vi "notification location.vi"(3 "Bottom Right":bool, 4 "Bottom Left":bool, 5 "Top Right":bool, 6 "Top Left":bool) -> (0 "ButtonStates":bool[](array[boolean]), 1 "Text Justification":enum16{"Left", "Center", "Right"}(ring), 2 "Position":T1)   [LabVIEW 2015]
uses:
  <vilib>/Utility/miscctls.llb/LVPositionTypeDef.ctl
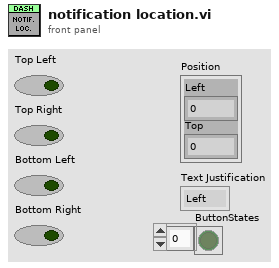
[diagram p1: front panel]
types:
  T1 = typedef "LVPositionTypeDef.ctl" = cluster{"Left":i32, "Top":i32}
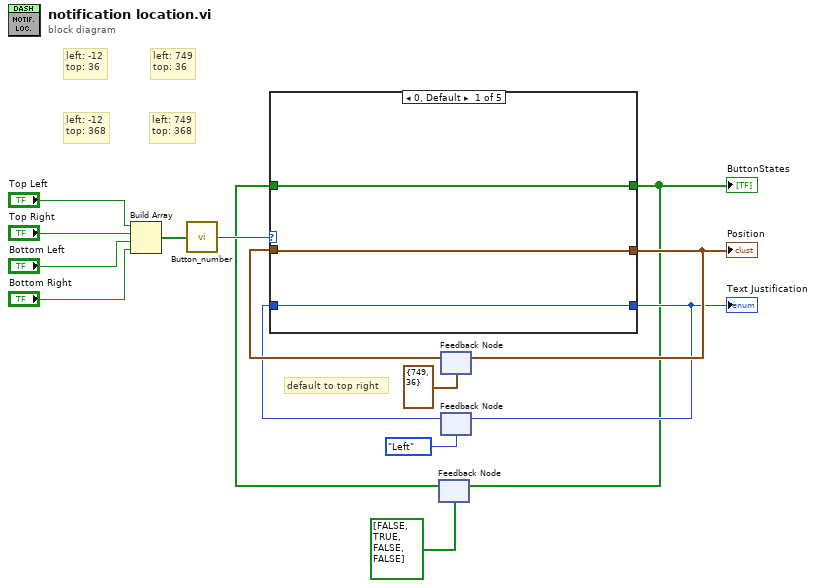
[diagram p0: block diagram]
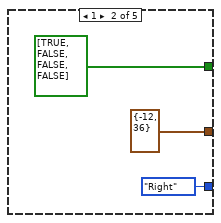
[diagram p2: hidden frame]
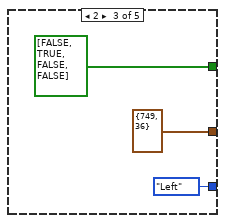
[diagram p3: hidden frame]
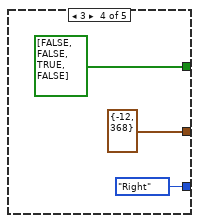
[diagram p4: hidden frame]
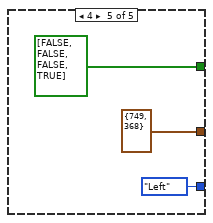
[diagram p5: hidden frame]
diagram:
  # "default to top right"
  # "left: -12\ntop: 368"
  # "left: -12\ntop: 36"
  # "left: 749\ntop: 368"
  # "left: 749\ntop: 36"
  n1 = Build Array("Top Left", "Top Right", "Bottom Left", "Bottom Right") -> (w11:bool[])
  n2 = call "Button_number.vi"("Button Array"=w11) -> ("Button Pressed"=w10:i32)
  n3 = feedback #1(bool[] [FALSE, TRUE, FALSE, FALSE]) -> (w2:bool[])
  n4 = feedback #2(T1 {"Left"=749, "Top"=36} ("Position")) -> (w7:T1)
  n5 = feedback #3(enum16{"Left", "Center", "Right"}."Left" ("Text.Justification")) -> (w5:enum16{"Left", "Center", "Right"})
  n6 = case shown="0, Default" w10 {
    tunnel: [w18 T1 {"Left"=-12, "Top"=36} ("Position") T1 {"Left"=749, "Top"=36} ("Position") T1 {"Left"=-12, "Top"=368} ("Position") T1 {"Left"=749, "Top"=368} ("Position")] -> w8
    tunnel: w7 -> [w18 _ _ _ _]
    tunnel: [w17 enum16{"Left", "Center", "Right"}."Right" ("Text.Justification") enum16{"Left", "Center", "Right"}."Left" ("Text.Justification") enum16{"Left", "Center", "Right"}."Right" ("Text.Justification") enum16{"Left", "Center", "Right"}."Left" ("Text.Justification")] -> w6
    tunnel: w5 -> [w17 _ _ _ _]
    tunnel: w2 -> [w16 _ _ _ _]
    tunnel: [w16 bool[] [TRUE, FALSE, FALSE, FALSE] bool[] [FALSE, TRUE, FALSE, FALSE] bool[] [FALSE, FALSE, TRUE, FALSE] bool[] [FALSE, FALSE, FALSE, TRUE]] -> w1
    frame 0, Default {
    }
    frame 1 {
    }
    frame 2 {
    }
    frame 3 {
    }
    frame 4 {
    }
  }
  "Position" <- w8
  "Text Justification" <- w6
  "ButtonStates" <- w1
  n7 = feedback-in #1(w1) -> ()
  n8 = feedback-in #2(w8) -> ()
  n9 = feedback-in #3(w6) -> ()
